vi "DMA.Scatter-Gather.Blocks to Block Descriptors.vi"(8 "error in (no error)":errorcluster, 11 "GE 5565PIORC":refnum<class "GE 5565PIORC.lvclass">) -> (0 "error out":errorcluster, 3 "GE 5565PIORC out":refnum<class "GE 5565PIORC.lvclass">)   [LabVIEW 2016, in "GE 5565PIORC.lvclass"]
uses:
  GE 5565PIORC.lvclass
  Controls/DMA Block.ctl
  Controls/DMA Block Descriptor.ctl
panel:
  out "Block Descriptors":T1[](array[typedef]) {"next descriptor ptr" format="%08x"; "data size" format="%08x"; "data ptr (upper)" format="%08x"; "data ptr (lower)" format="%08x"; "descriptor ptr (aligned)" format="%08x"; "descriptor size" format="%08x"; "descriptor ptr (VISA)" format="%08x"}
  in  "Blocks":T2[](array[typedef]) {"size" format="%08x"; "pointer" format="%08x"}
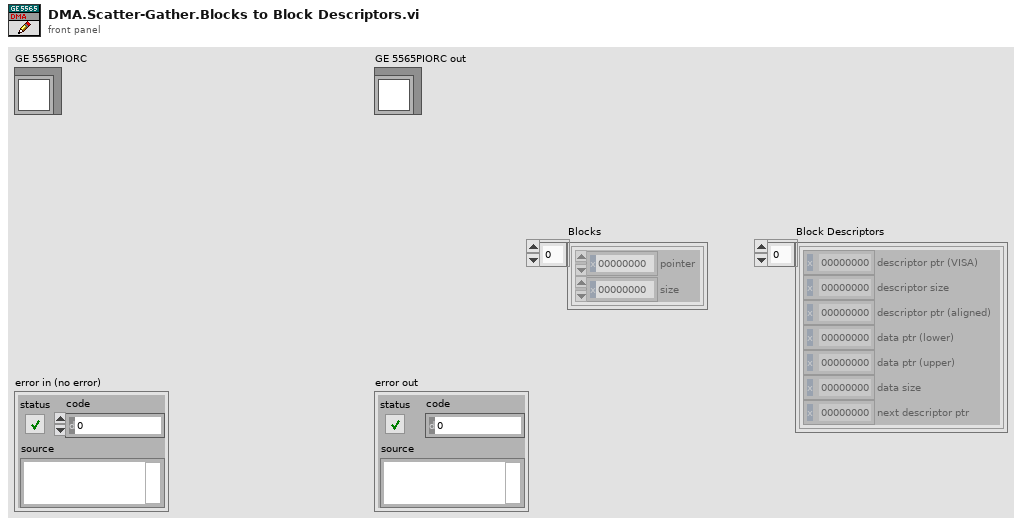
[diagram p1: front panel]
types:
  T1 = typedef "GE 5565PIORC.lvclass/DMA Block Descriptor.ctl" = cluster{"descriptor ptr (VISA)":u32, "descriptor size":u32, "descriptor ptr (aligned)":u32, "data ptr (lower)":u32, "data ptr (upper)":u32, "data size":u32, "next descriptor ptr":u32}
  T2 = typedef "GE 5565PIORC.lvclass/DMA Block.ctl" = cluster{"pointer":u32, "size":u32}
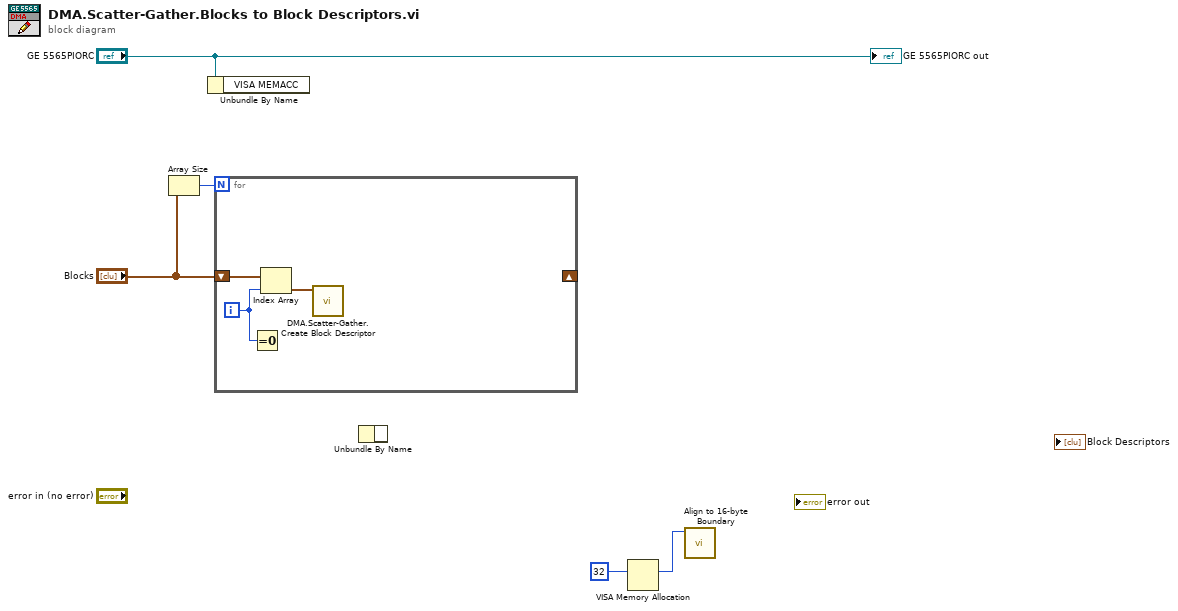
[diagram p0: block diagram]
diagram:
  n1 = Array Size(array="Blocks") -> (size(s)=w1:i32)
  n2 = Unbundle By Name("GE 5565PIORC") -> ()  [unwired: 1 out]
  n3 = for {
    N: w1 -> [_]
    shift-right: _ -> [_]
    shift-left: "Blocks" -> [w8]
    i -> [w7]
    n4 = Equal To 0?(x=w7) -> ()  [unwired: 1 out]
    n5 = Index Array(array=w8, index=w7) -> (element=w6:T2)
    n6 = call "DMA.Scatter-Gather.Create Block Descriptor.vi"("block"=w6) -> ()  [unwired: 10 in, 1 out]
  }
  n7 = Unbundle By Name() -> ()  [unwired: 1 in, 1 out]
  n8 = VISA Memory Allocation(10:u32 32 ("size")) -> (2:w3:u32)  [unwired: 2 in, 2 out]
  n9 = call "Align to 16-byte Boundary.vi"("pointer"=w3) -> ()  [unwired: 10 in, 1 out]
  "GE 5565PIORC out" <- "GE 5565PIORC"
